vi "PIStageInit.vi"(1 "error in (no error)":errorcluster) -> (0 "error out":errorcluster)   [LabVIEW 2009]
uses:
  StageSettings.ctt
  <vilib>/Utility/config.llb/NI_LVConfig.lvlib
panel:
  out "PI Stage Setup":T1={"channels (x, y, z)"="2", "Stage Scaling (V/µm)"=0.1} {"Stage Scaling (V/µm)" format="%.2f"}
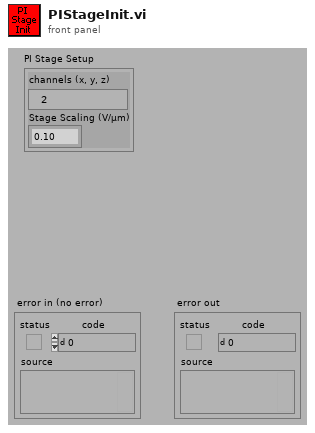
[diagram p1: front panel]
types:
  T1 = typedef "StageSettings.ctt" = cluster{"channels (x, y, z)":tag, "Stage Scaling (V/µm)":dbl}
  T2 = typedef "NI_LVConfig.lvlib/Config Data RefNum.ctl" = refnum<k1>
  T3 = cluster{"channels (x, y, z)":tag, "Stage Scaling (V/µm)":dbl}
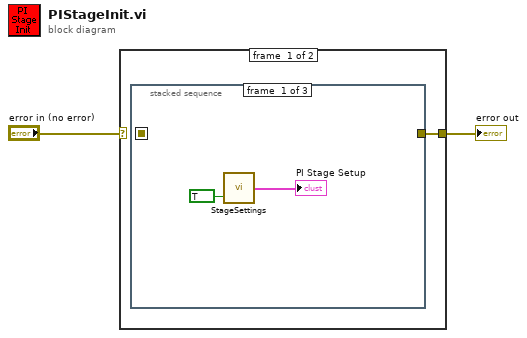
[diagram p0: block diagram]
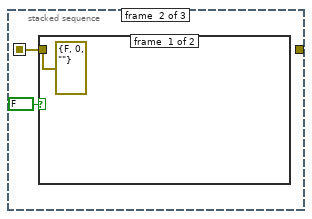
[diagram p2: hidden frame]
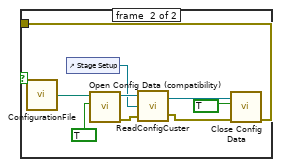
[diagram p3: hidden frame]
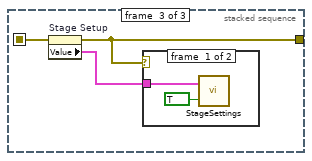
[diagram p4: hidden frame]
diagram:
  n1 = case shown="No Error" "error in (no error)" {
    selector: "error in (no error)" -> [_ w23]
    tunnel: [w3 w23] -> w1
    frame #0 {
      n2 = stacked-sequence {
        seq-local: [_ w7 _] -> [_ _ w20]
        tunnel: [_ _ w19] -> w3
        frame #0 {
          n3 = call "StageSettings.vi"("Get/Set"=TRUE) -> ("PI Stage Setup (output)"=→"PI Stage Setup":T1)  [unwired: 1 in]
        }
        frame #1 {
          n4 = case shown="False" FALSE {
            tunnel: [errorcluster {"status"=FALSE, "code"=0, "source"=""} ("error out") w13] -> w7
            frame #0 {
            }
            frame #1 {
              n5 = call "ConfigurationFile.vi"() -> ("Configuration File (output)"=w12:path)  [unwired: 2 in]
              n6 = control-ref of="Stage Setup"() -> (w11:refnum<vi>)
              n7 = call <vilib>:"Open Config Data (compatibility).vi"("create file if necessary (T)"=TRUE ("create file if necessary? (T)"), "configuration file path"=w12) -> ("error out"=w15:errorcluster, "refnum"=w16:T2)  [unwired: 7 in, 1 out]
              n8 = call "ReadConfigCuster.vi"("error in (no error)"=w15, "Ctrl Reference"=w11, "ConfigFile (input)"=w16) -> ("error out"=w9:errorcluster, "ConfigFile (output)"=w10:T2)
              n9 = call "Close Config Data.vi"("error in (no error)"=w9, "write configuration file? (T)"=TRUE ("write configuration file? (F)"), "refnum"=w10) -> ("error out"=w13:errorcluster)  [unwired: 8 in]
            }
          }
        }
        frame #2 {
          n10 = property on="Stage Setup" class="Clust (strict)"(error in=w20) -> (error out=w19:errorcluster, "Value"=w18:T3)  [unwired: 1 in, 1 out]
          n11 = case shown="No Error" w19 {
            tunnel: w18 -> [w21 _]
            frame #0 {
              n12 = call "StageSettings.vi"("Get/Set"=TRUE ("Set"), "PI Stage Setup (input)"=w21) -> ()  [unwired: 1 out]
            }
            frame #1 {
            }
          }
        }
      }
    }
    frame #1 {
    }
  }
  "error out" <- w1
